vi "OverlayPAReport.vi"(7 "Group":string, 8 "error in":errorcluster, 9 "Color":u32(colorbox)=16711680, 10 "Particle Reports (Pixels)":T1(array[cluster]) {"Orientation" format="%.2f"; "Dimensions"."Height" format="%.2f"; "Dimensions"."Width" format="%.2f"; "Center of Mass"."Y" format="%.2f"; "Center of Mass"."X" format="%.2f"; "Bounding Rect"."Bottom" format="%.2f"; "Bounding Rect"."Right" format="%.2f"; "Bounding Rect"."Top" format="%.2f"; "Bounding Rect"."Left" format="%.2f"; "Number of Holes" format="%.2f"; "Area" format="%.2f"}, 11 "Image":T2) -> (0 "error out":errorcluster, 3 "Image Out":T2)   [LabVIEW 2016]
doc: "Overlay targets at the location of the feature points in the specified colors."
uses:
  <vilib>/vision/Image Controls.llb/IMAQ Image.ctl
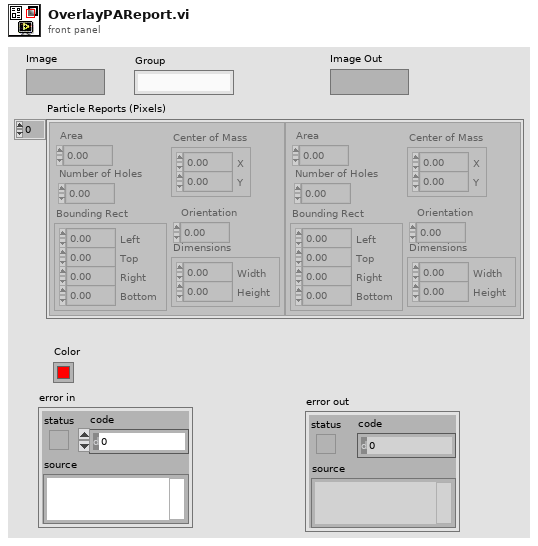
[diagram p1: front panel]
types:
  T1 = cluster{"Area":dbl, "Number of Holes":dbl, "Bounding Rect":cluster{"Left":dbl, "Top":dbl, "Right":dbl, "Bottom":dbl}, "Center of Mass":cluster{"X":dbl, "Y":dbl}, "Orientation":dbl, "Dimensions":cluster{"Width":dbl, "Height":dbl}}[]
  T2 = typedef "IMAQ Image.ctl" = refnum<image>
  T3 = cluster{"Left":dbl, "Top":dbl, "Right":dbl, "Bottom":dbl}
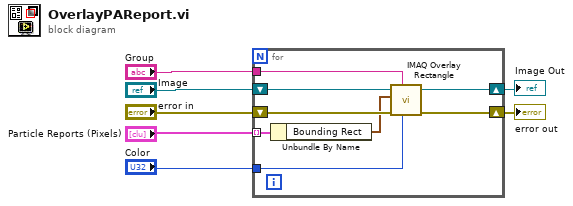
[diagram p0: block diagram]
diagram:
  n1 = for {
    tunnel: "Particle Reports (Pixels)" -> [w9] mode=indexing
    tunnel: "Group" -> [w14]
    tunnel: "Color" -> [w11]
    shift-right: [w10] -> w7
    shift-left: "Image" -> [w15]
    shift-right: [w12] -> w3
    shift-left: "error in" -> [w13]
    n2 = Unbundle By Name(w9) -> ("Bounding Rect"=w8:T3)
    n3 = call "IMAQ Overlay Rectangle"("Color"=w11, "Group"=w14, "error in (no error)"=w13, "Rectangle"=w8, "Image"=w15) -> ("error out"=w12:errorcluster, "Image Out"=w10:T2)  [unwired: 5 in]
  }
  "Image Out" <- w7
  "error out" <- w3
